vi "Get Status Event.vi"(8 "error in (no error)":errorcluster, 11 "Status in":refnum<class "Status.lvclass">) -> (0 "error out":errorcluster, 2 "Status Event":refnum<user-event>, 3 "Status out":refnum<class "Status.lvclass">)   [LabVIEW 2020, in "neg-pkg.lvlib" / "Status.lvclass"]
uses:
  Status.lvclass
  Status Message Data.ctl
  Status.lvclass/Status.ctl
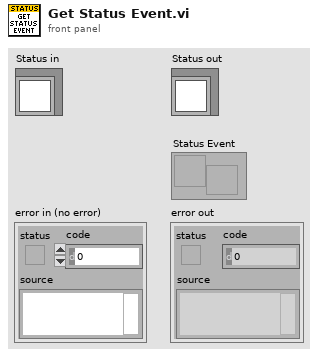
[diagram p1: front panel]
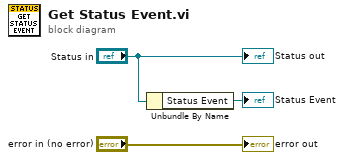
[diagram p0: block diagram]
diagram:
  n1 = Unbundle By Name("Status in") -> ("Status Event"=→"Status Event":refnum<user-event>)
  "error out" <- "error in (no error)"
  "Status out" <- "Status in"
